vi "Initialize dynamic image handling.vi"(10 "Camera label mapping":T1(array[cluster]), 11 "Inspection.Image details_init":T2(array[cluster])) -> (1 "ISIM":u8[](array[numeric]), 2 "Combined camera names":string[](array[string]), 3 "Image indicator labels":string[](array[string]))   [LabVIEW 2019, in "ZenGage v3.0 UI.lvclass"]
uses:
  ZenGage v3.0 UI.lvclass
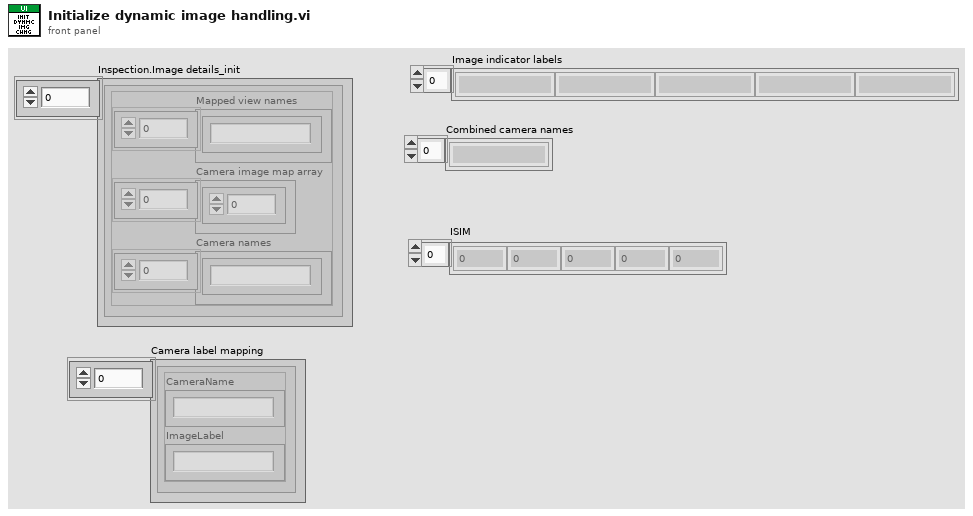
[diagram p1: front panel]
types:
  T1 = cluster{"CameraName":string, "ImageLabel":string}[]
  T2 = cluster{"Mapped view names":string[], "Camera image map array":i32[], "Camera names":string[]}[]
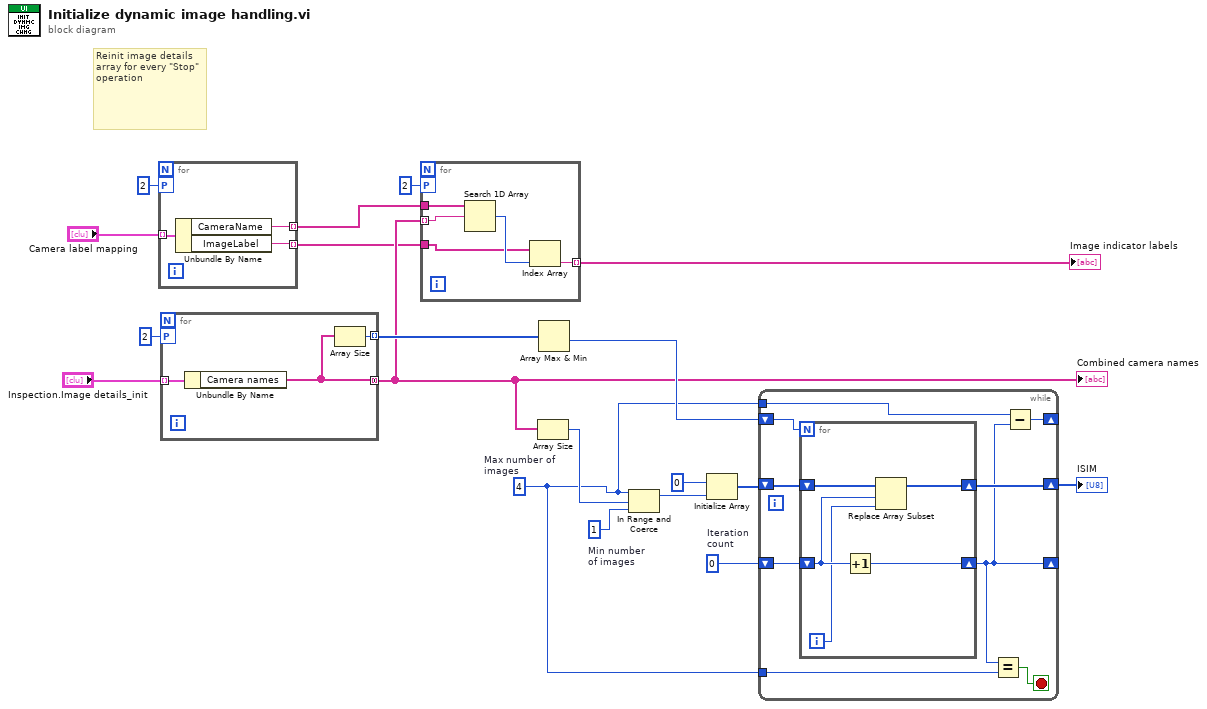
[diagram p0: block diagram]
diagram:
  w11 = 0  # Iteration count
  w17 = 1  # Min number of images
  w9 = 4  # Max number of  images
  # "Reinit image details\narray for every \"Stop\" operation"
  n1 = for {
    tunnel: "Camera label mapping" -> [w22] mode=indexing
    tunnel: [w21] -> w6 mode=indexing
    tunnel: [w20] -> w5 mode=indexing
    workers-P: 2 -> [_]
    n2 = Unbundle By Name(w22) -> ("CameraName"=w21:string, "ImageLabel"=w20:string)
  }
  n3 = for {
    tunnel: "Inspection.Image details_init" -> [w25] mode=indexing
    tunnel: [w24] -> w7 mode=concatenating
    tunnel: [w23] -> w13 mode=indexing
    workers-P: 2 -> [_]
    n4 = Unbundle By Name(w25) -> ("Camera names"=w24:string[])
    n5 = Array Size(array=w24) -> (size(s)=w23:i32)
  }
  "Combined camera names" <- w7
  n6 = for {
    tunnel: w7 -> [w29] mode=indexing
    tunnel: w6 -> [w30]
    tunnel: w5 -> [w27]
    tunnel: [w26] -> w4 mode=indexing
    workers-P: 2 -> [_]
    n7 = Search 1D Array(1D array=w30, element=w29) -> (index of element=w28:i32)  [unwired: 1 in]
    n8 = Index Array(array=w27, index=w28) -> (element=w26:string)
  }
  "Image indicator labels" <- w4
  n9 = Array Size(array=w7) -> (size(s)=w18:i32)
  n10 = Array Max & Min(array=w13) -> (min value=w12:i32)  [unwired: 3 out]
  n11 = In Range and Coerce(upper limit=w9, x=w18, lower limit=w17) -> (coerced(x)=w16:i32)  [unwired: 1 out]
  n12 = Initialize Array(u8 0, w16) -> (w14:u8[])
  n13 = while {
    shift-right: [w32] -> _
    shift-left: w11 -> [w36]
    tunnel: w9 -> [w35]
    tunnel: w9 -> [w33]
    shift-right: [w31] -> _
    shift-left: w12 -> [w37]
    shift-right: [w38] -> w10
    shift-left: w14 -> [w39]
    stop <- w34 stop-if-true
    n14 = for {
      N: w37 -> [_]
      shift-right: [w43] -> w38
      shift-left: w39 -> [w44]
      shift-right: [w42] -> w32
      shift-left: w36 -> [w41]
      i -> [w40]
      n15 = Increment(x=w41) -> (x+1=w42:i32)
      n16 = Replace Array Subset(array=w44, new element=w40, index=w41) -> (w43:u8[])
    }
    n17 = Equal?(x=w32, y=w35) -> (x = y?=w34:bool)
    n18 = Subtract(x=w33, y=w32) -> (x-y=w31:i32)
  }
  "ISIM" <- w10
